vi "doesnanonissuck.vi"() -> ()   [LabVIEW 2019]
uses:
  <userlib>/Nanonis Prog Interface V5/Nanonis Prog Interface.lvlib
panel:
  out "time for execution":u32
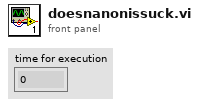
[diagram p1: front panel]
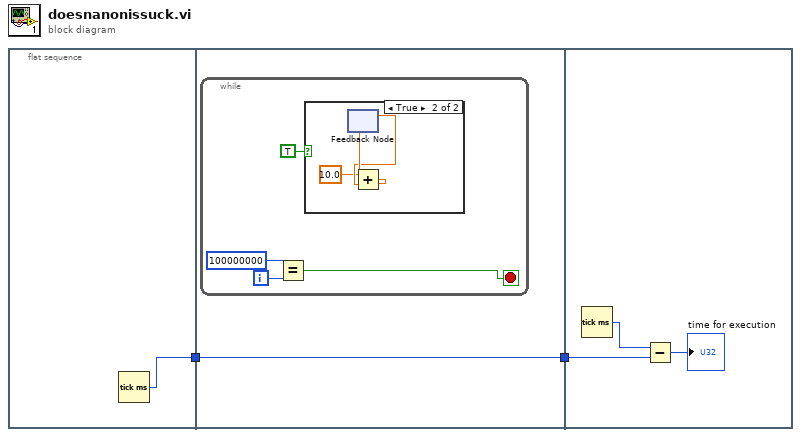
[diagram p0: block diagram]
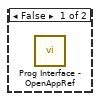
[diagram p2: hidden frame]
diagram:
  n1 = flat-sequence {
    tunnel: [w3] -> w2
    tunnel: w2 -> [w4]
    tunnel: [w4] -> w1
    tunnel: w1 -> [w13]
    frame #0 {
      n2 = Tick Count (ms)() -> (millisecond timer value=w3:u32)
    }
    frame #1 {
      n3 = while {
        i -> [w8]
        stop <- w6 stop-if-true
        n4 = Equal?(x=100000000, y=w8) -> (x = y?=w6:bool)
        n5 = case shown="True" TRUE {
          frame False {
            n6 = call <userlib>:"Prog Interface - OpenAppRef.vi"() -> ()  [unwired: 6 in, 2 out]
          }
          frame True {
            n7 = feedback #1() -> (w10:dbl)  [unwired: 1 in]
            n8 = Add(x=10.0, y=w10) -> (x+y=w11:dbl)
            n9 = feedback-in #1(w11) -> ()
          }
        }
      }
    }
    frame #2 {
      n10 = Tick Count (ms)() -> (millisecond timer value=w14:u32)
      n11 = Subtract(x=w14, y=w13) -> (x-y=→"time for execution":u32)
    }
  }
